vi "Error Message.vi"() -> (2 "Error":string)   [LabVIEW 2015]
uses:
  Galobal variable_TI.vi
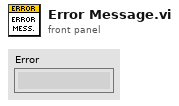
[diagram p1: front panel]
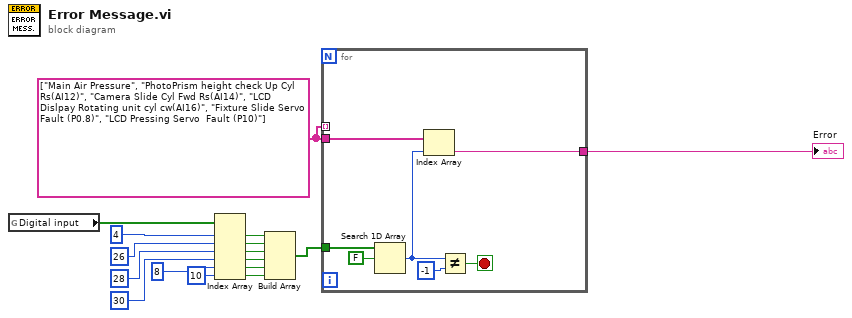
[diagram p0: block diagram]
diagram:
  w7 = string[] ["Main Air Pressure", "PhotoPrism height check Up Cyl Rs(AI12)", "Camera Slide Cyl Fwd Rs(AI14)", "LCD Dislpay Rotating unit cyl cw(AI16)", "Fixture Slide Servo Fault (P0.8)", "LCD Pressing Servo  Fault (P10)"]
  n1 = global read "Galobal variable_TI.vi" "Digital input"() -> (w16:bool[])
  n2 = Index Array(array=w16, index #1=4 ("index"), index #2=26 ("index"), index #3=28 ("index"), index #4=30 ("index"), index #5=8 ("index"), index #6=10 ("index")) -> (element #1=w11:bool, element #2=w10:bool, element #3=w9:bool, element #4=w8:bool, element #5=w2:bool, element #6=w1:bool)
  n3 = Build Array(w11, w10, w9, w8, w2, w1) -> (w6:bool[])
  n4 = for {
    tunnel: w7 -> [_] mode=indexing
    tunnel: w7 -> [w19]
    tunnel: w6 -> [w21]
    tunnel: [w17] -> w5
    stop <- w20 stop-if-true
    n5 = Search 1D Array(1D array=w21, element=FALSE) -> (index of element=w18:i32)  [unwired: 1 in]
    n6 = Index Array(array=w19, index=w18) -> (element=w17:string)
    n7 = Not Equal?(x=w18, y=-1) -> (x != y?=w20:bool)
  }
  "Error" <- w5
